vi "FTP Send Whole Directory.vi"(8 "timeout ms (60000)":i32=200, 10 "Local Folder of Autonomous Plays":path, 11 "host":string="10.26.14.21") -> (0 "error out":errorcluster)   [LabVIEW 2016]
uses:
  <vilib>/FTP/NI_FTP.lvlib
panel:
  out "error out 2":errorcluster
  out "Array":T1(array[cluster])
  in  "Target Remote directory path":string="/Autonomous-Plays"
  in  "password":string
  in  "user":string="anonymous"
  out "file errors":errorcluster[](array[cluster])
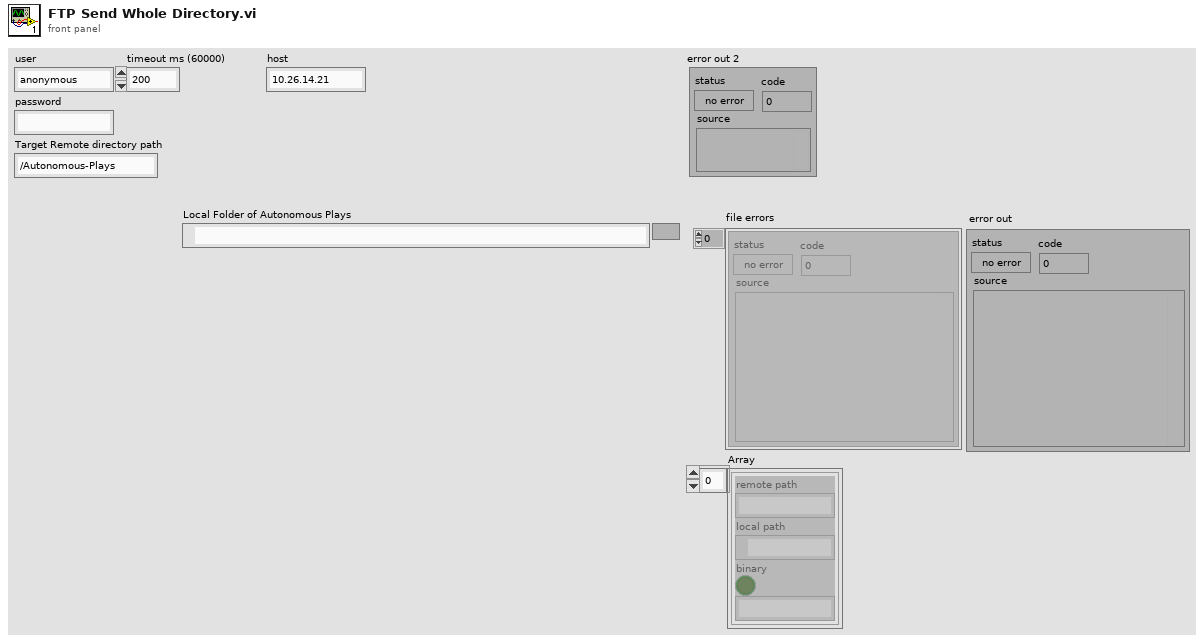
[diagram p1: front panel]
types:
  T1 = cluster{"remote path":string, "local path":path, "binary":bool, string}[]
  T2 = cluster{"remote path":string, "local path":path, "binary":bool, string}
  T3 = typedef "NI_FTP.lvlib/FTP Session.ctl" = refnum<k5>
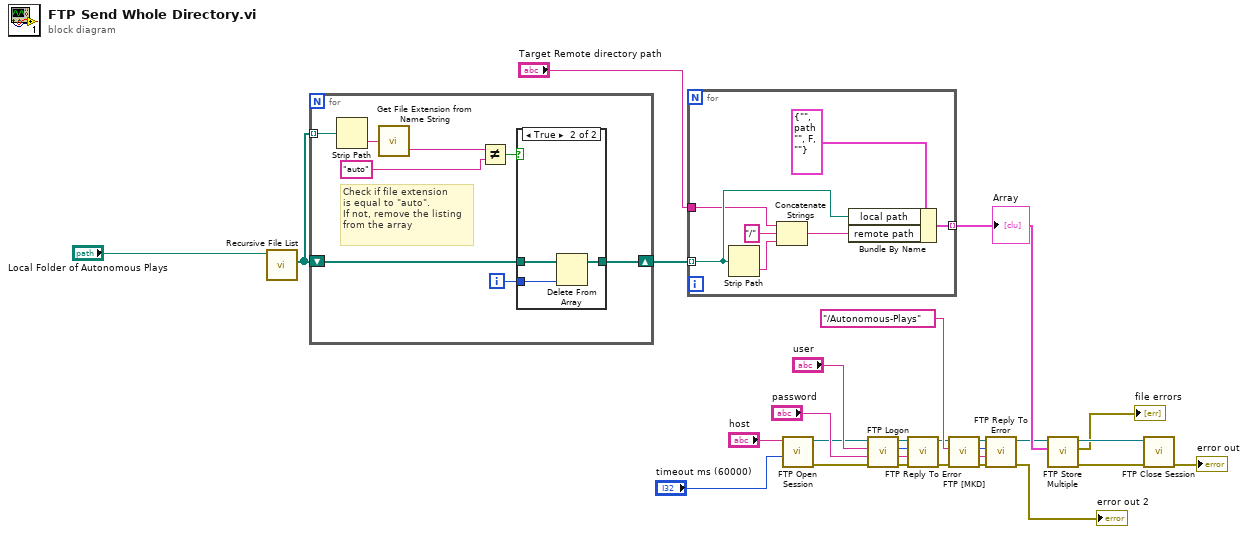
[diagram p0: block diagram]
diagram:
  n1 = call <vilib>:"Recursive File List.vi"("Folder Path"="Local Folder of Autonomous Plays") -> ("All Files in Dir"=w28:path[])  [unwired: 6 in, 4 out]
  n2 = for {
    tunnel: w28 -> [w31] mode=indexing
    shift-right: [w29] -> w26
    shift-left: w28 -> [w35]
    i -> [w33]
    # "Check if file extension\nis equal to \"auto\".\nIf not, remove the listing\nfrom the array"
    n3 = Strip Path(path=w31) -> (name=w30:string)  [unwired: 1 out]
    n4 = call "Get File Extension from Name String.vi"("File Name String"=w30) -> ("lowercase file extension"=w32:string)  [unwired: 1 out]
    n5 = Not Equal?(x=w32, y="auto") -> (x != y?=w34:bool)
    n6 = case shown="True" w34 {
      tunnel: w35 -> [w37 w39]
      tunnel: w33 -> [_ w40]
      tunnel: [w37 w38] -> w29
      frame False {
      }
      frame True {
        n7 = Delete From Array(array=w39, index=w40) -> (array with subset deleted=w38:path[])  [unwired: 1 in, 1 out]
      }
    }
  }
  n8 = for {
    tunnel: w26 -> [w46] mode=indexing
    tunnel: "Target Remote directory path" -> [w45]
    tunnel: [w41] -> w20 mode=indexing
    n9 = Strip Path(path=w46) -> (name=w43:string)  [unwired: 1 out]
    n10 = Concatenate Strings(w45, "/" ("string"), w43) -> (w42:string)
    n11 = Bundle By Name(cluster=T2 {"remote path"="", "local path"=path "", "binary"=FALSE, ""} ("transfer spec"), "local path"=w46, "remote path"=w42) -> (w41:T2)
  }
  "Array" <- w20
  n12 = call <vilib>:"FTP Open Session.vi"("timeout ms (60000)"="timeout ms (60000)", "address"="host") -> ("error out"=w17:errorcluster, "ftp session"=w18:T3)  [unwired: 6 in, 2 out]
  n13 = call <vilib>:"FTP Logon.vi"("error in (no error)"=w17, "password"="password", "user"="user", "ftp session"=w18) -> ("error out"=w9:errorcluster, "reply string"=w10:string, "reply code"=w11:i32, "ftp session out"=w12:T3)  [unwired: 4 in]
  n14 = call <vilib>:"FTP Reply To Error.vi"("error in (no error)"=w9, "reply string in"=w10, "reply code in"=w11, "ftp session"=w12) -> ("error out"=w8:errorcluster, "ftp session out"=w7:T3)  [unwired: 2 out]
  n15 = call <vilib>:"FTP [MKD].vi"("error in (no error)"=w8, "directory path"="/Autonomous-Plays", "ftp session"=w7) -> ("error out"=w3:errorcluster, "reply string"=w4:string, "reply code"=w5:i32, "ftp session out"=w6:T3)  [unwired: 5 in]
  n16 = call <vilib>:"FTP Reply To Error.vi"("error in (no error)"=w3, "reply string in"=w4, "reply code in"=w5, "ftp session"=w6) -> ("error out"=→"error out 2":errorcluster, "ftp session out"=w2:T3)  [unwired: 2 out]
  n17 = call <vilib>:"FTP Store Multiple.vi"("file specifications"=w20, "ftp session"=w2) -> ("error out"=w15:errorcluster, "file errors"=→"file errors":errorcluster[], "ftp session out"=w16:T3)  [unwired: 7 in]
  n18 = call <vilib>:"FTP Close Session.vi"("error in (no error)"=w15, "ftp session"=w16) -> ("error out"=→"error out":errorcluster)  [unwired: 6 in, 3 out]
